vi "Geneate_Model_Name.vi"(11 "Model_Info_and_Report":T1 {"Rel_Margin" format="%#.5f"; "Bad_Min(Img)" format="%#.5f"; "Good_Max(Img)" format="%#.5f"; "Pixel_F1_Max" format="%#.5f"; "Pixel_AUC" format="%#.5f"; "Image_F1_Max" format="%#.5f"; "Image_AUC" format="%#.5f"}) -> (3 "Model_Name":string)   [LabVIEW 2020]
uses:
  Controls/Model_Info_and_Report.ctl
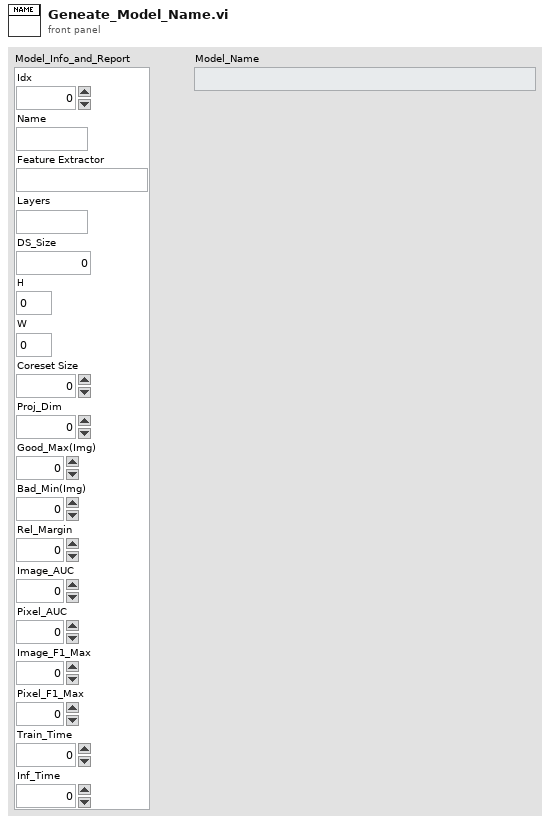
[diagram p1: front panel]
types:
  T1 = typedef "Model_Info_and_Report.ctl" = cluster{"Idx":i32, "Name":string, "Feature Extractor":string, "Layers":string, "DS_Size":i32, "H":i32, "W":i32, "Coreset Size":i32, "Proj_Dim":i32, "Good_Max(Img)":sgl, "Bad_Min(Img)":sgl, "Rel_Margin":sgl, "Image_AUC":sgl, "Pixel_AUC":sgl, "Image_F1_Max":sgl, "Pixel_F1_Max":sgl, "Train_Time":dbl, "Inf_Time":dbl}
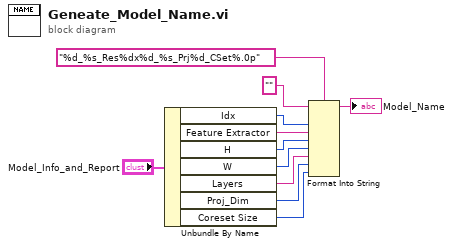
[diagram p0: block diagram]
diagram:
  n1 = Unbundle By Name("Model_Info_and_Report") -> ("Idx"=w4:i32, "Feature Extractor"=w6:string, "H"=w3:i32, "W"=w2:i32, "Layers"=w1:string, "Proj_Dim"=w8:i32, "Coreset Size"=w7:i32)
  n2 = Format Into String(format string="%d_%s_Res%dx%d_%s_Prj%d_CSet%.0p", initial string="", w4, w6, w3, w2, w1, w8, w7) -> (resulting string=→"Model_Name":string)  [unwired: 1 in, 1 out]
